vi "Set Default Policy Version.vi"(8 "error in (no error)":errorcluster, 9 "Version":i32, 10 "Name":string, 11 "IoT Session in":refnum<class "IoT Session.lvclass">) -> (0 "error out":errorcluster, 3 "IoT Session out":refnum<class "IoT Session.lvclass">)   [LabVIEW 2015, in "NI_AWS_IoT.lvlib" / "IoT Session.lvclass"]
uses:
  IoT Session.lvclass
  Core/HTTP Request/Request Options.ctl
  Core/HTTP Request/Name Value Pair.ctl
  Core/HTTP Request/Region handling.ctl
  Core/HTTP Request/URL formatting.ctl
  Core/HTTP Request/HTTP Request.lvclass
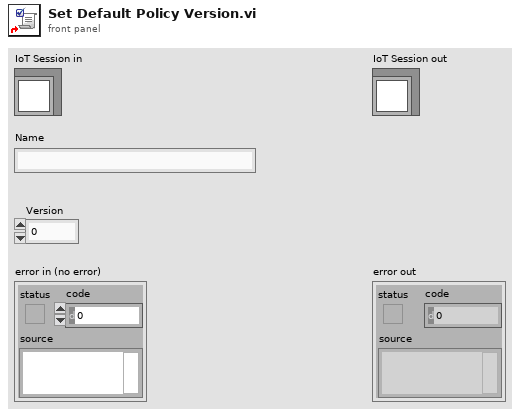
[diagram p1: front panel]
types:
  T1 = typedef "NI_AWS_Core.lvlib/HTTP Request.lvclass/Name Value Pair.ctl" = cluster{"name":string, "value":string}
  T2 = typedef "NI_AWS_Core.lvlib/HTTP Request.lvclass/Request Options.ctl" = cluster{"request headers":T1[], "request parameters":T1[], "request body":string, "region handling":T3, "URL formatting":T4}
  T3 = typedef "NI_AWS_Core.lvlib/HTTP Request.lvclass/Region handling.ctl" = enum16{"use region everywhere", "use region (authentication only)", "use region (URL only)", "ignore region everwhere"}
  T4 = typedef "NI_AWS_Core.lvlib/HTTP Request.lvclass/URL formatting.ctl" = enum16{"region-", "region."}
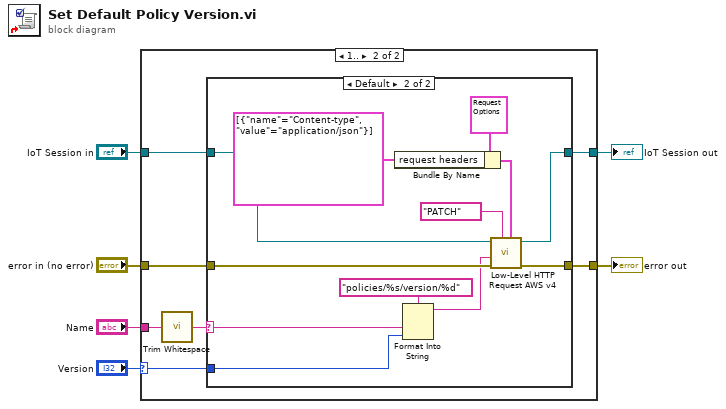
[diagram p0: block diagram]
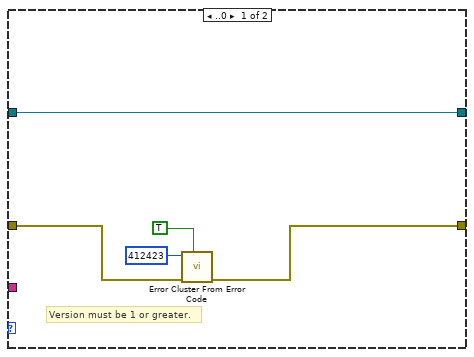
[diagram p2: hidden frame]
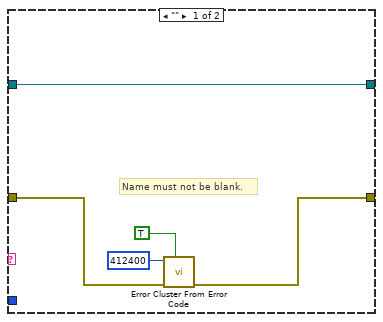
[diagram p3: hidden frame]
diagram:
  n1 = case shown="1.." "Version" {
    selector: "Version" -> [_ w13]
    tunnel: "error in (no error)" -> [w8 w18]
    tunnel: [w7 w17] -> w5
    tunnel: [w11 w16] -> w4
    tunnel: "IoT Session in" -> [w11 w15]
    tunnel: "Name" -> [_ w14]
    frame ..0 {
      # "Version must be 1 or greater."
      n2 = call <vilib>:"Error Cluster From Error Code.vi"("show call chain? (False)"=TRUE, "error in (no error)"=w8, "error code (0)"=412423) -> ("error out"=w7:errorcluster)  [unwired: 6 in]
    }
    frame 1.. {
      n3 = call <vilib>:"Trim Whitespace.vi"("string"=w14) -> ("trimmed string"=w12:string)  [unwired: 1 in]
      n4 = case shown="Default" w12 {
        selector: w12 -> [_ w26]
        tunnel: w18 -> [w21 w35]
        tunnel: [w20 w34] -> w17
        tunnel: [w19 w33] -> w16
        tunnel: w15 -> [w19 w32]
        tunnel: w13 -> [_ w25]
        frame "" {
          # "Name must not be blank."
          n5 = call <vilib>:"Error Cluster From Error Code.vi"("show call chain? (False)"=TRUE, "error in (no error)"=w21, "error code (0)"=412400) -> ("error out"=w20:errorcluster)  [unwired: 6 in]
        }
        frame Default {
          n6 = Bundle By Name(cluster=T2 {"request headers"=[], "request parameters"=[], "request body"="", "region handling"=enum."use region everywhere", "URL formatting"=enum."region."} ("Request Options"), "request headers"=T1[] [{"name"="Content-type", "value"="application/json"}]) -> (w30:T2)
          n7 = Format Into String(format string="policies/%s/version/%d" ("string"), w26, w25) -> (resulting string=w28:string)  [unwired: 2 in, 1 out]
          n8 = call "Low-Level HTTP Request AWS v4.vi"("Request Options"=w30, "HTTP-Verb"="PATCH", "error in (no error)"=w35, "URL Suffix"=w28, "AWS Core in"=w32) -> ("error out"=w34:errorcluster, "AWS Core out"=w33:refnum<class "IoT Session.lvclass">)  [unwired: 3 in, 2 out]
        }
      }
    }
  }
  "error out" <- w5
  "IoT Session out" <- w4
